vi "Write NewParameters.vi"(8 "error in (no error)":errorcluster, 10 "NewParameters":T1={"PenaltyDistance"=0.0, "DistanceAttackerToBackBall"=0.0, "Division"=enum."Div B", "DistanceToAvoidyEnemyRobot"=0.0, "BallPlacementDistance"=900.0, "DisatanceBehindBallToStealBall"=0.0, "MaxDistanceToPositionKickoff"=2000.0, "BlockEnemyTarget"=FALSE, "MaxStopVAng"=1.0, "DistanceMarkerToEnemy"=0.0, "IgnoreDribblerContact"=FALSE, "DistanceToBeginEnemyPosession"=200.0, "GoToBallWhenEnemyNotMoving"=TRUE, "EnemyDistanceToReduceVelocity"=500.0, "TurnOnEnemyDistanceToReduceVelocity"=TRUE, "EnemyDistanceToShootOutBall"=500.0, "DefenseKickBall"=TRUE, "MoreKickToGoal? (0-0.3)"=0.0, "ChipKickInEnemyField"=TRUE, "ShootOutRobotId"=0.0, "FieldLenghtDenominatorInShootOut"=0.0, "AdjustPositionInBallPlacement"=FALSE, "PowerGodPass"=0.0, "VelocityAbortEnemyPos"=0.0, "MaxDistToBeginPass"=500.0, "MinDistToBeginPass"=150.0, "VelocityInDirects"=0.3, "BadDribblerIDs"=[], "NewKickToDistanceAroundBall"=300.0, "PowerAvoidColisionMarker"=0.5, "DistanceToAvoidColisionMarker"=250.0, "AvoidBallKick"=0.0, "DistanceTryKick"=0.0, "SuicideKickDIstance"=0.0, "AdjustFirstKickDistance"=0.0, "AvoidAimLessKick"=0.0, "DistanceToAvoidyEnemyShootRobot "=0.0, "NumberOfMarkers"=3.0, "PotField"=TRUE, "PIDLateral"=FALSE, "MinDistanceFirstKickX"=0.0, "MinDistanceFirstKickY"=0.0, "FractionOfDistToTouchGround\nAfterChipKick"=0.8, "FractionOfKickxWhen\nComposedWithKickz"=0.0, "Style"=enum."Insanity", "MoveInTurnState"=TRUE, "DistFromEnemyToConsider\nMoveInTurnState"=0.0, "CascadePID"=TRUE, "TurnAroundParameters"={"Radius"=0.0, "Multiplier"=0.0, "ChordAngle"=0.0}, "SafeDriveVel"=0.5, "DistanceToGoToBackBall"=500.0, "minDistanceToNotFinish\nEnemyPossession"=0.0, "OneTouchShot"={"angleFactor"=0.0, "maxAngle"=0.0, "Attack"=FALSE, "Defense"=FALSE}, "OpenAngleToGoal"={"minAngle"=0.0, "maxAngle"=0.0, "minEvaluation"=0.0}, "ShotInterception"={"shotSpeed"=0.0, "minEnemySpeed"=0.0, "maxEnemySpeed"=0.0, "minEvaluation"=0.0}, "AllyTeamArray"=[], "maxDefendersNumber"=0, "Zone"={"GuardPositionArray"=[], "ZoneMidField"=[], "CenterForwardWidth"=0.0}, "MinEvaluationToShoot"=0.0, "PassInterception"={"maxPassSpeed"=0.0, "minPassSpeed"=0.0, "minEnemySpeed"=0.0, "chipPassDistance"=0.0, "chipPassEvaluation"=0.0, "minEvaluation"=0.0, "maxEnemySpeed"=0.0}, "PassDistance"={"maxDistance"=0.0, "minDistance"=0.0}, "receiverSpeed"=0.0, "maxBallSpeed"=0.0, "slackTime"=0.0, "Turning radius"=0.0, "Turning v_ang"=0.0, "AlignError"={"Distance"=0.0, "Orientation"=0.0, "V_norm(m/s)"=0.0, "V_ang (rad/s)"=0.0}, "RobotRadius"=0.0, "KickerDistance"=0.0, "keeper angle  to cover goalpost"=0.0}, 11 "Game in":refnum<class "Game.lvclass">) -> (0 "error out":errorcluster, 3 "Game out":refnum<class "Game.lvclass">)   [LabVIEW 2023, in "Game.lvclass"]
uses:
  Game.lvclass
  Controls/NewParameters.ctl
  Utilities_class/Style.ctl
  Controls/AllyTeam.ctl
  Game.lvclass/Game.ctl
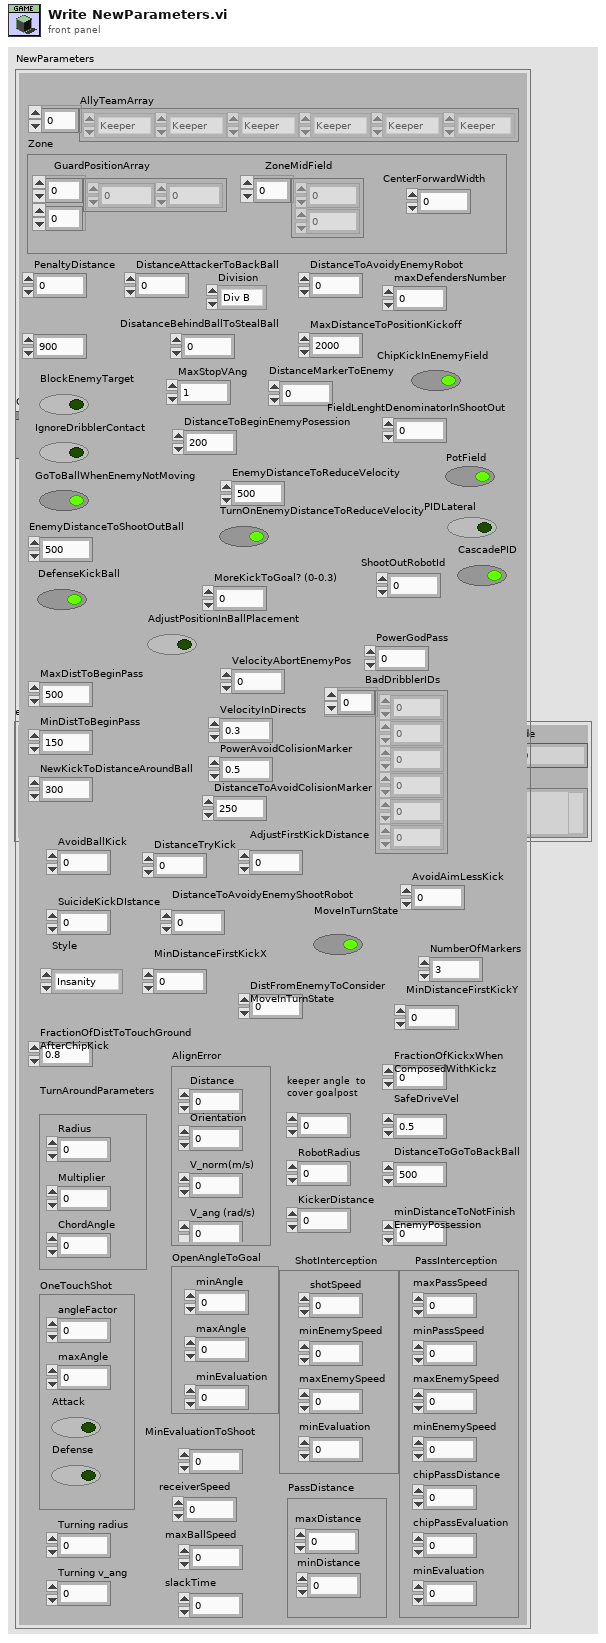
[diagram p1: front panel]
types:
  T1 = typedef "NewParameters.ctl" = cluster{"PenaltyDistance":dbl, "DistanceAttackerToBackBall":dbl, "Division":enum16{"Div B", "Div A"}, "DistanceToAvoidyEnemyRobot":dbl, "BallPlacementDistance":dbl, "DisatanceBehindBallToStealBall":dbl, "MaxDistanceToPositionKickoff":dbl, "BlockEnemyTarget":bool, "MaxStopVAng":dbl, "DistanceMarkerToEnemy":dbl, "IgnoreDribblerContact":bool, "DistanceToBeginEnemyPosession":dbl, "GoToBallWhenEnemyNotMoving":bool, "EnemyDistanceToReduceVelocity":dbl, "TurnOnEnemyDistanceToReduceVelocity":bool, "EnemyDistanceToShootOutBall":dbl, "DefenseKickBall":bool, "MoreKickToGoal? (0-0.3)":dbl, "ChipKickInEnemyField":bool, "ShootOutRobotId":dbl, "FieldLenghtDenominatorInShootOut":dbl, "AdjustPositionInBallPlacement":bool, "PowerGodPass":dbl, "VelocityAbortEnemyPos":dbl, "MaxDistToBeginPass":dbl, "MinDistToBeginPass":dbl, "VelocityInDirects":dbl, "BadDribblerIDs":i32[], "NewKickToDistanceAroundBall":dbl, "PowerAvoidColisionMarker":dbl, "DistanceToAvoidColisionMarker":dbl, "AvoidBallKick":dbl, "DistanceTryKick":dbl, "SuicideKickDIstance":dbl, "AdjustFirstKickDistance":dbl, "AvoidAimLessKick":dbl, "DistanceToAvoidyEnemyShootRobot ":dbl, "NumberOfMarkers":dbl, "PotField":bool, "PIDLateral":bool, "MinDistanceFirstKickX":dbl, "MinDistanceFirstKickY":dbl, "FractionOfDistToTouchGround\nAfterChipKick":dbl, "FractionOfKickxWhen\nComposedWithKickz":dbl, "Style":T2, "MoveInTurnState":bool, "DistFromEnemyToConsider\nMoveInTurnState":dbl, "CascadePID":bool, "TurnAroundParameters":cluster{"Radius":dbl, "Multiplier":dbl, "ChordAngle":dbl}, "SafeDriveVel":dbl, "DistanceToGoToBackBall":dbl, "minDistanceToNotFinish\nEnemyPossession":dbl, "OneTouchShot":cluster{"angleFactor":dbl, "maxAngle":dbl, "Attack":bool, "Defense":bool}, "OpenAngleToGoal":cluster{"minAngle":dbl, "maxAngle":dbl, "minEvaluation":dbl}, "ShotInterception":cluster{"shotSpeed":dbl, "minEnemySpeed":dbl, "maxEnemySpeed":dbl, "minEvaluation":dbl}, "AllyTeamArray":T3[], "maxDefendersNumber":i32, "Zone":cluster{"GuardPositionArray":dbl[][], "ZoneMidField":dbl[], "CenterForwardWidth":dbl}, "MinEvaluationToShoot":dbl, "PassInterception":cluster{"maxPassSpeed":dbl, "minPassSpeed":dbl, "minEnemySpeed":dbl, "chipPassDistance":dbl, "chipPassEvaluation":dbl, "minEvaluation":dbl, "maxEnemySpeed":dbl}, "PassDistance":cluster{"maxDistance":dbl, "minDistance":dbl}, "receiverSpeed":dbl, "maxBallSpeed":dbl, "slackTime":dbl, "Turning radius":dbl, "Turning v_ang":dbl, "AlignError":cluster{"Distance":dbl, "Orientation":dbl, "V_norm(m/s)":dbl, "V_ang (rad/s)":dbl}, "RobotRadius":dbl, "KickerDistance":dbl, "keeper angle  to cover goalpost":dbl}
  T2 = typedef "Style.ctl" = enum16{"Insanity", "Offensive", "Defensive"}
  T3 = typedef "AllyTeam.ctl" = enum16{"Keeper", "Defender", "Attacker"}
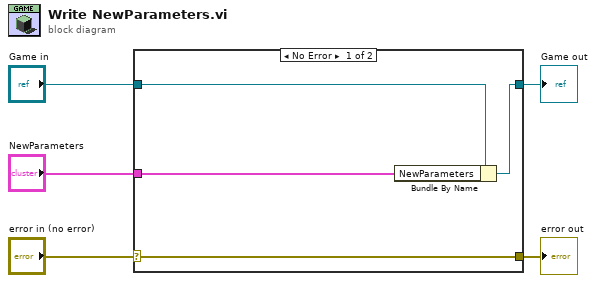
[diagram p0: block diagram]
diagram:
  n1 = case shown="No Error" "error in (no error)" {
    selector: "error in (no error)" -> [w9 w10]
    tunnel: [w9 w10] -> w4
    tunnel: [w7 w11] -> w2
    tunnel: "Game in" -> [w8 w11]
    tunnel: "NewParameters" -> [w6 _]
    frame No Error {
      n2 = Bundle By Name(cluster=w8, "NewParameters"=w6) -> (w7:refnum<class "Game.lvclass">)
    }
    frame Error {
    }
  }
  "error out" <- w4
  "Game out" <- w2
